vi "Clear Min ROI Overlay.vi"(8 "error in (no error)":errorcluster, 11 "Image in":T1) -> (0 "error out":errorcluster, 3 "Image out":T1)   [LabVIEW 2011, in "Meter Detection Custom Device.lvlib"]
uses:
  Meter Detection Custom Device.lvlib
  <vilib>/vision/Image Controls.llb/IMAQ Image.ctl
  Shared/Meter Detection Global Variable.vi
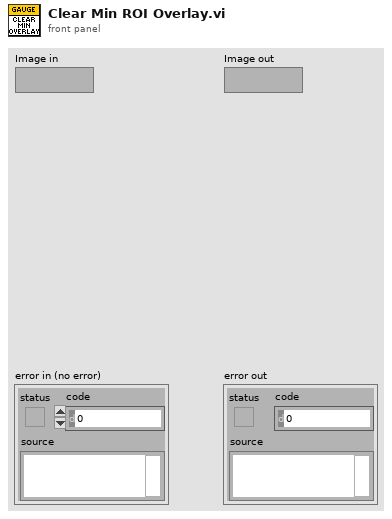
[diagram p1: front panel]
types:
  T1 = typedef "IMAQ Image.ctl" = refnum<image>
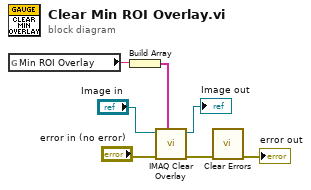
[diagram p0: block diagram]
diagram:
  n1 = global read "Meter Detection Global Variable.vi" "Min ROI Overlay"() -> (w7:string)
  n2 = Build Array(w7) -> (w6:string[])
  n3 = call "IMAQ Clear Overlay"("Groups"=w6, "error in (no error)"="error in (no error)", "Image"="Image in") -> ("error out"=w2:errorcluster, "Image Out"=→"Image out":T1)  [unwired: 7 in]
  n4 = call <vilib>:"Clear Errors.vi"("error in (no error)"=w2) -> ("error out"=→"error out":errorcluster)  [unwired: 6 in]
